vi "tm_setshadingframe.vi"(8 "error in (no error)":errorcluster, 9 "Frame":i32(ring)=1 items=["Frame 1"=1, "Frame 2"=2, "Frame 3"=3, "Frame 4"=4], 10 "Enable":bool, 11 "Handle in":u32) -> (0 "error out":errorcluster, 3 "Handle out":u32)   [LabVIEW 2012]
uses:
  tmcamcon.dll
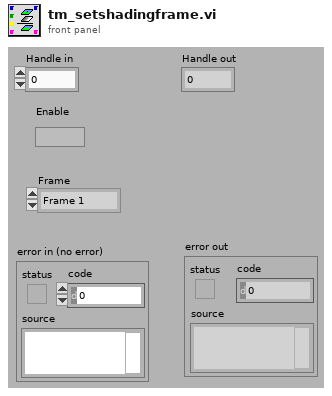
[diagram p1: front panel]
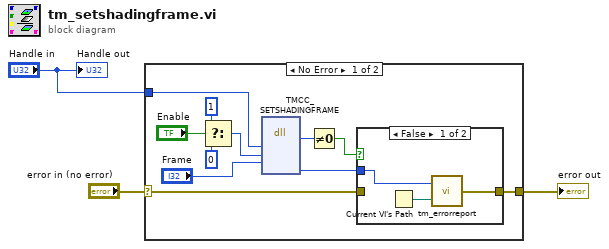
[diagram p0: block diagram]
diagram:
  n1 = case shown="No Error" "error in (no error)" {
    selector: "error in (no error)" -> [w7 w19]
    tunnel: [w4 w19] -> w2
    tunnel: "Handle in" -> [w8 _]
    frame No Error {
      n2 = Select(t=1, s="Enable", f=0) -> (s? t:f=w9:i32)
      n3 = dll-call lib="tmcamcon.dll" fn="TMCC_SETSHADINGFRAME"("Handle"=w8, "enable"=w9, "frame"="Frame") -> ("return type"=w14:u32, "Erval"=w6:i32)  [unwired: 7 in, 2 out]
      n4 = Not Equal To 0?(x=w14) -> (x != 0?=w5:bool)
      n5 = case shown="False" w5 {
        tunnel: w7 -> [_ w18]
        tunnel: [w16 w18] -> w4
        tunnel: w6 -> [w15 _]
        frame False {
          n6 = Current VI's Path() -> (path=w17:path)
          n7 = call "tm_errorreport.vi"("Source"=w17, "Error"=w15) -> ("error out"=w16:errorcluster)
        }
        frame True {
        }
      }
    }
    frame Error {
    }
  }
  "error out" <- w2
  "Handle out" <- "Handle in"
